vi "Event from Boolean.vi"(7 "Time Stamp":timestamp, 9 "Name":string, 10 "Value":bool, 11 "VI Refnum":refnum<vi>) -> (2 "Event Data":T1)   [LabVIEW 2023, in "Instruments.lvlib" / "Instruments.lvclass"]
uses:
  Library/Instruments.lvclass
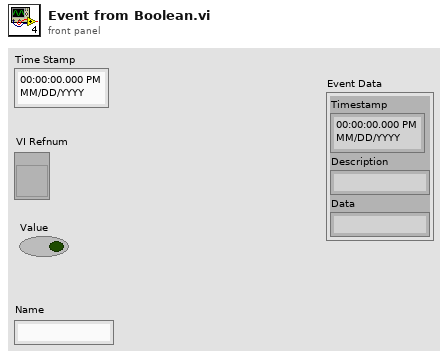
[diagram p1: front panel]
types:
  T1 = cluster{"Timestamp":timestamp, "Description":string, "Data":string}
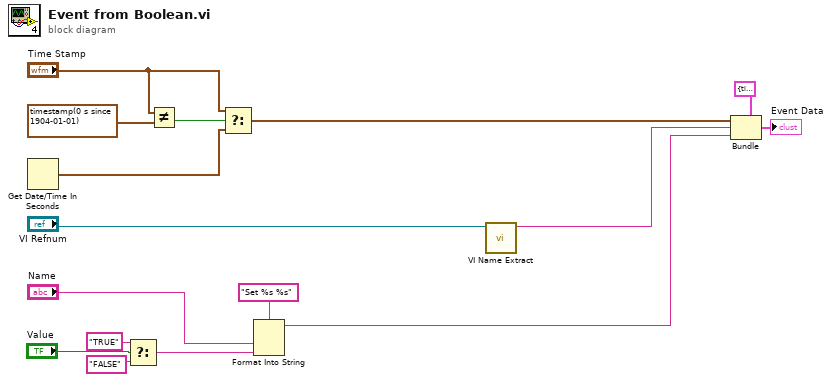
[diagram p0: block diagram]
diagram:
  n1 = Get Date/Time In Seconds() -> (seconds since 1Jan1904=w11:timestamp)
  n2 = Select(t="TRUE", s="Value", f="FALSE") -> (s? t:f=w3:string)
  n3 = Not Equal?(x="Time Stamp", y=timestamp(0 s since 1904-01-01) ("Time Stamp")) -> (x != y?=w13:bool)
  n4 = Select(t="Time Stamp", s=w13, f=w11) -> (s? t:f=w10:timestamp)
  n5 = Format Into String(format string="Set %s %s", "Name", w3) -> (resulting string=w8:string)  [unwired: 2 in, 1 out]
  n6 = call "VI Name Extract.vi"("VI Refnum"="VI Refnum") -> ("Name"=w1:string)  [unwired: 10 in]
  n7 = Bundle(cluster=T1 {"Timestamp"=timestamp(0 s since 1904-01-01), "Description"="", "Data"=""}, "Timestamp"=w10, "Description"=w1, "Data"=w8) -> (→"Event Data":T1)
